vi "CloseCollection.vi"(8 "error in (no error)":errorcluster, 11 "MongoDB-Collection in":refnum<class "MongoDB-Collection.lvclass">) -> (0 "error out":errorcluster)   [LabVIEW 2016, in "MongoDB-Collection.lvlib" / "MongoDB-Collection.lvclass"]
uses:
  MongoDB-Collection.lvclass
  D:/Users/blume/Desktop/LV/MongoDB-Driver/MLV DLLs/MongoLabVIEW.dll
  LV/MongoDB-Driver/MLV DLLs/MongoLabVIEW.dll
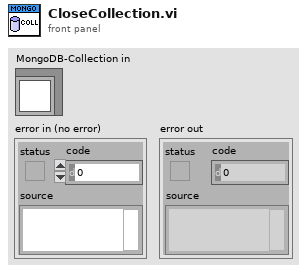
[diagram p1: front panel]
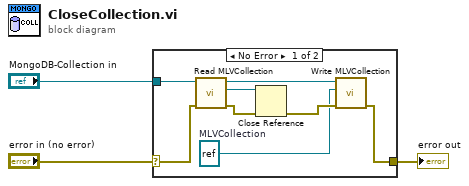
[diagram p0: block diagram]
diagram:
  n1 = case shown="No Error" "error in (no error)" {
    selector: "error in (no error)" -> [w10 w12]
    tunnel: [w4 w12] -> w2
    tunnel: "MongoDB-Collection in" -> [w11 _]
    frame No Error {
      w5 = refnum<k24> refnum  # MLVCollection
      n2 = call "Read MLVCollection.vi"("error in (no error)"=w10, "MongoDB-Collection in"=w11) -> ("error out"=w8:errorcluster, "MLVCollection"=w9:refnum<k24>, "MongoDB-Collection out"=w7:refnum<class "MongoDB-Collection.lvclass">)  [unwired: 7 in]
      n3 = Close Reference(reference=w9, error in (no error)=w8) -> (error out=w6:errorcluster)
      n4 = call "Write MLVCollection.vi"("error in (no error)"=w6, "MLVCollection"=w5, "MongoDB-Collection in"=w7) -> ("error out"=w4:errorcluster)  [unwired: 7 in, 1 out]
    }
    frame Error {
    }
  }
  "error out" <- w2
